vi "Espera notificacion.vi"() -> ()   [LabVIEW 2019]
panel:
  out "Numeric":i32
  out "notification":string
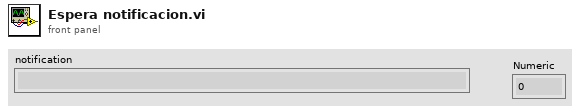
[diagram p1: front panel]
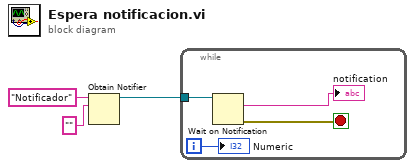
[diagram p0: block diagram]
diagram:
  n1 = Obtain Notifier(name (unnamed)="Notificador", notification data type="") -> (notifier out=w2:refnum<notifier>)  [unwired: 2 in, 2 out]
  n2 = while {
    tunnel: w2 -> [w5]
    i -> [w4]
    stop <- w7 stop-if-true
    n3 = Wait on Notification(notifier=w5) -> (notification=→"notification":string, error out=w7:errorcluster)  [unwired: 3 in, 2 out]
    "Numeric" <- w4
  }
